vi "gyro measurement.vi"() -> ()   [LabVIEW 2015]
uses:
  <vilib>/Analysis/baseanly.llb/Mean (DBL).vi
  <vilib>/Analysis/NI_AALBase.lvlib
panel:
  out "Waveform Chart 2":dbl(graph)
  out "Waveform Chart":dbl(graph)
  out "mean":dbl format="%0.2f"
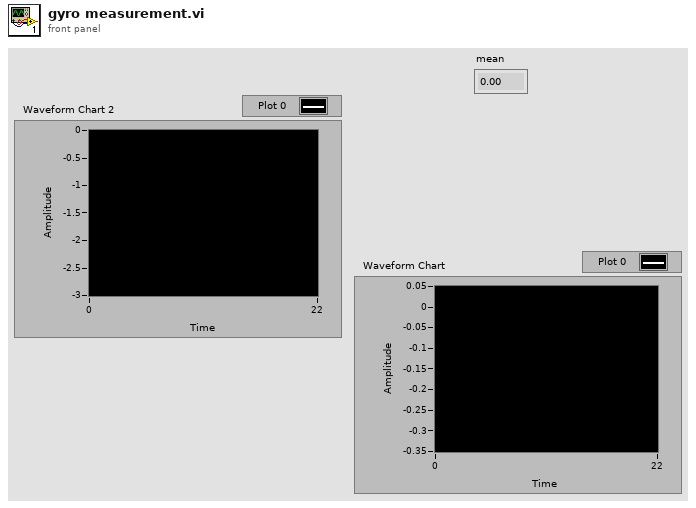
[diagram p1: front panel]
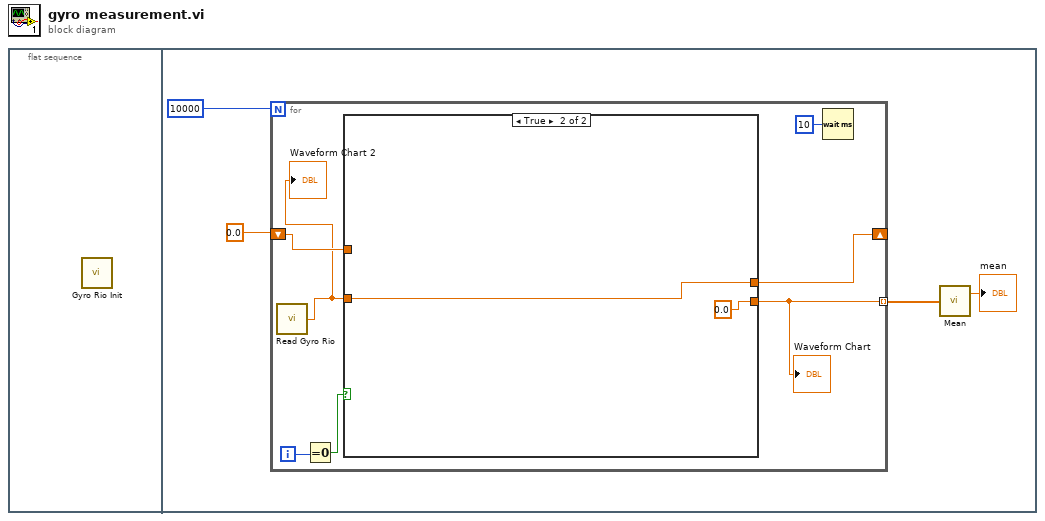
[diagram p0: block diagram]
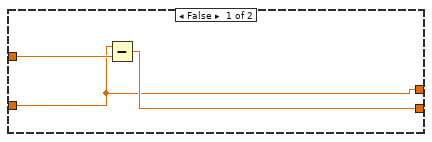
[diagram p2: hidden frame]
diagram:
  n1 = flat-sequence {
    frame #0 {
      n2 = call "Gyro Rio Init.vi"() -> ()  [unwired: 12 in]
    }
    frame #1 {
      n3 = for {
        N: 10000 -> [_]
        shift-right: [w9] -> _
        shift-left: 0.0 -> [w8]
        tunnel: [w6] -> w3 mode=indexing
        i -> [w10]
        n4 = call "Read Gyro Rio.vi"() -> ("integral y(t)"=w5:dbl)  [unwired: 1 in, 2 out]
        "Waveform Chart 2" <- w5
        n5 = Equal To 0?(x=w10) -> (x = 0?=w7:bool)
        n6 = case shown="True" w7 {
          tunnel: [w12 w16] -> w9
          tunnel: w5 -> [w12 w16]
          tunnel: w8 -> [w14 _]
          tunnel: [w13 0.0] -> w6
          frame False {
            n7 = Subtract(x=w12, y=w14) -> (x-y=w13:dbl)
          }
          frame True {
          }
        }
        "Waveform Chart" <- w6
        n8 = Wait (ms)(milliseconds to wait=u32 10) -> ()  [unwired: 1 out]
      }
      n9 = call-poly <vilib>:"Mean.vi"("X"=w3) -> ("mean"=→"mean":dbl)  [unwired: 1 out]
    }
  }
